vi "from string array.vi"(8 "error in (no error)":errorcluster, 9 "String Array":string[][](array[string]), 10 "version":string, 11 "module configuration in":refnum<class "SystemLink File configuration.lvclass">) -> (0 "error out":errorcluster, 3 "module configuration out":refnum<class "SystemLink File configuration.lvclass">)   [LabVIEW 2015]
uses:
  <vilib>/NI/Tag Bus Module Framework/channel/TBM channel.lvclass
  SystemLink File configuration.lvclass
  permissions.ctl
  Line.ctl
  Data Tag Type.ctl
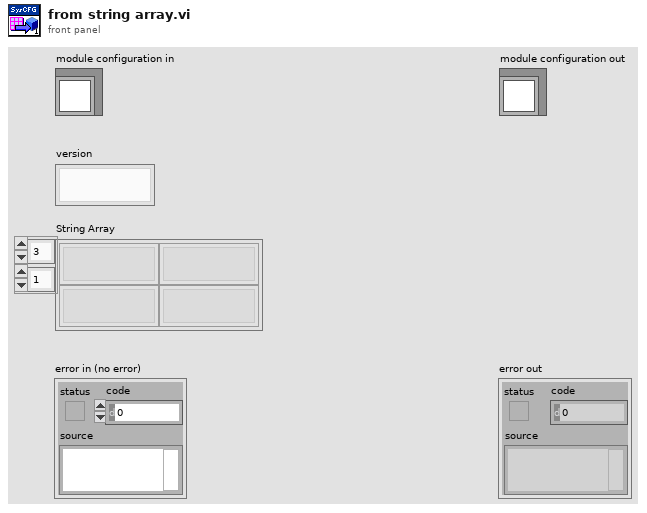
[diagram p1: front panel]
types:
  T1 = typedef "SystemLink File configuration.lvclass/Data Tag Type.ctl" = enum16{"Double", "Single", "I32", "I16", "I8", "U64", "U32", "U16", "U8", "Boolean", "String", "Timestamp"}
  T2 = typedef "SystemLink File configuration.lvclass/Line.ctl" = cluster{"channel":refnum<class "TBM channel.lvclass">, "Data Tag Type":T1}
  T3 = typedef "SystemLink File configuration.lvclass/permissions.ctl" = enum32{"Read from SystemLink", "Write to SystemLink"}
  T4 = typedef "tag bus.lvlib/tag descriptor.lvclass/Data Type.ctl" = enum16{"Double", "Single", "I64", "I32", "I16", "I8", "U64", "U32", "U16", "U8", "Boolean", "String", "Array of Double", "Array of Single", "Array of I64", "Array of I32", "Array of I16", "Array of I8", "Array of U64", "Array of U32", "Array of U16", "Array of U8", "Array of Boolean", "Array of String"}
  T5 = typedef "TBM channel.lvclass/channel classification.ctl" = enum16{"input data", "output data", "processing parameter", "processing result"}
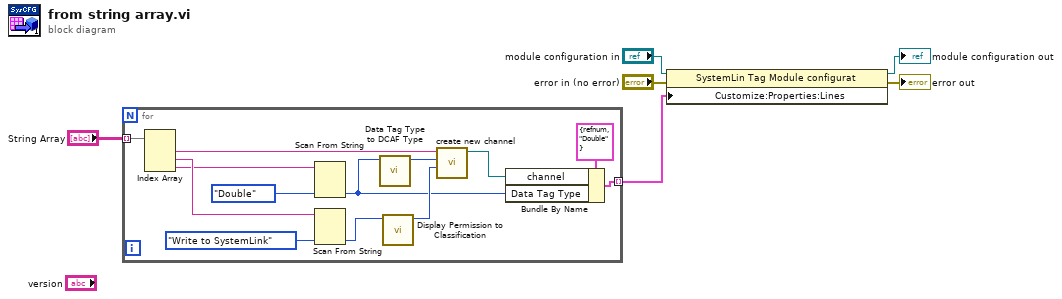
[diagram p0: block diagram]
diagram:
  n1 = for {
    tunnel: "String Array" -> [w19] mode=indexing
    tunnel: [w10] -> w1 mode=indexing
    n2 = Index Array(array=w19) -> (element #1=w18:string, element #2=w14:string, element #3=w13:string)  [unwired: 3 in]
    n3 = Scan From String(input string=w13, default 1=Data_Tag_Type."Double" ("Data Tag Type")) -> (output 1=w7:T1)  [unwired: 3 in, 3 out]
    n4 = Scan From String(input string=w14, default 1=permissions."Write to SystemLink" ("display permissions")) -> (output 1=w16:T3)  [unwired: 3 in, 3 out]
    n5 = call "Data Tag Type to DCAF Type.vi"("Data Tag Type"=w7) -> ("DCAF Data Type"=w8:T4)  [unwired: 10 in]
    n6 = call "Display Permission to Classification.vi"("display permissions"=w16) -> ("channel classification"=w15:T5)  [unwired: 10 in]
    n7 = call <vilib>:"create new channel.vi"("channel classification"=w15, "data type"=w8, "channel name"=w18) -> ("channel"=w11:refnum<class "TBM channel.lvclass">)  [unwired: 8 in]
    n8 = Bundle By Name(cluster=T2 {"channel"=refnum, "Data Tag Type"=enum."Double"} ("Line"), "channel"=w11, "Data Tag Type"=w7) -> (w10:T2)
  }
  n9 = property class="SystemLin Tag Module configurat"(reference="module configuration in", error in="error in (no error)", "Customize:Properties:Lines"=w1) -> (reference out=→"module configuration out":refnum<class "SystemLink File configuration.lvclass">, error out=→"error out":errorcluster)
